vi "OpenVeriStandConnection.vi"(6 "Gateway IP Address (\"\": localhost)":string, 7 "Minimum VeriStand Version (2016)":string="2016", 8 "error in (no error)":errorcluster, 9 "overrides files":path[](array[path]), 10 "System Definition File":path, 11 "VeriStand Test Case in":refnum<class "VeriStandTestCase.lvclass">) -> (0 "error out":errorcluster, 1 "Open Skipped":bool, 3 "VeriStand Test Case out":refnum<class "VeriStandTestCase.lvclass">)   [LabVIEW 2027, in "VeriStandTestCase.lvclass"]
uses:
  VeriStandTestCase.lvclass
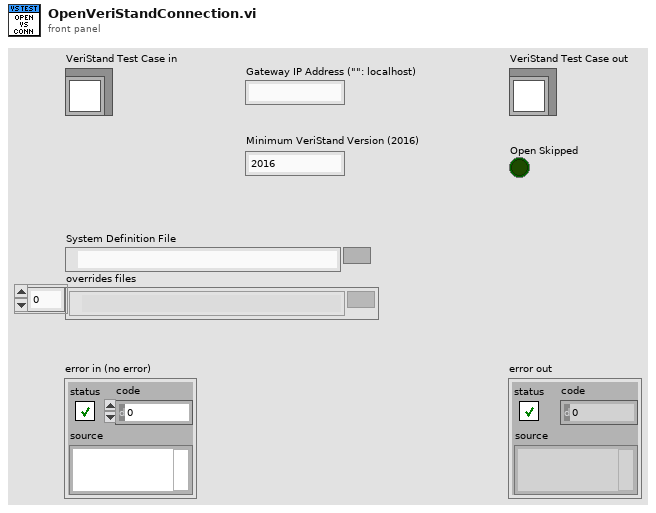
[diagram p1: front panel]
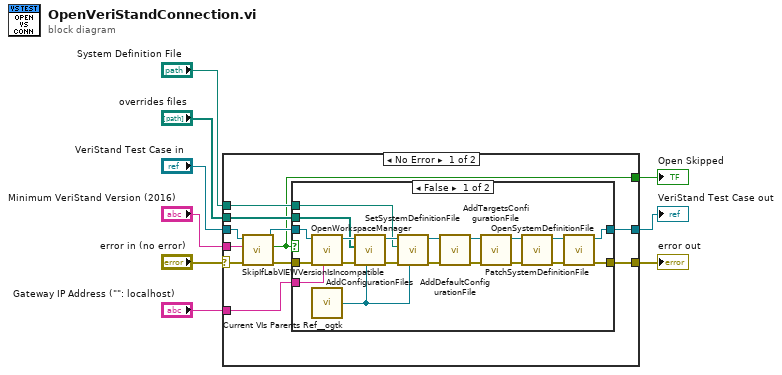
[diagram p0: block diagram]
diagram:
  n1 = case shown="No Error" "error in (no error)" {
    selector: "error in (no error)" -> [w13 w44]
    tunnel: [w19 w44] -> w8
    tunnel: [w20 w43] -> w6
    tunnel: "VeriStand Test Case in" -> [w15 w43]
    tunnel: "System Definition File" -> [w17 _]
    tunnel: "Gateway IP Address (\"\": localhost)" -> [w18 _]
    tunnel: "overrides files" -> [w16 _]
    tunnel: "Minimum VeriStand Version (2016)" -> [w14 _]
    tunnel: [w10 _] -> w1
    frame No Error {
      n2 = call "SkipIfLabVIEWVersionIsIncompatible.vi"("error in (no error)"=w13, "Minimum Version Year (2016)"=w14, "VeriStandTestCase in"=w15) -> ("error out"=w12:errorcluster, "Skipped"=w10:bool, "VeriStandTestCase out"=w11:refnum<class "VeriStandTestCase.lvclass">)  [unwired: 6 in]
      n3 = case shown="False" w10 {
        tunnel: [w40 w42] -> w20
        tunnel: [w39 w41] -> w19
        tunnel: w18 -> [w38 _]
        tunnel: w17 -> [w27 _]
        tunnel: w16 -> [w31 _]
        tunnel: w11 -> [w35 w42]
        tunnel: w12 -> [w34 w41]
        frame False {
          n4 = call "OpenWorkspaceManager.vi"("Gateway IP Address (\"\": localhost)"=w38, "error in (no error)"=w34, "VeriStandTestCase in"=w35) -> ("error out"=w32:errorcluster, "VeriStandTestCase out"=w33:refnum<class "VeriStandTestCase.lvclass">)  [unwired: 7 in]
          n5 = call <userlib>:"Current VIs Parents Ref__ogtk.vi"() -> ("Calling VI's Reference"=w28:refnum<vi>)  [unwired: 2 in]
          n6 = call "AddConfigurationFiles.vi"("path root vi ref (calling vi)"=w28, "error in (no error)"=w32, "configuration files"=w31, "VeriStandTestCase in"=w33) -> ("error out"=w29:errorcluster, "VeriStandTestCase out"=w30:refnum<class "VeriStandTestCase.lvclass">)  [unwired: 6 in]
          n7 = call "SetSystemDefinitionFile.vi"("path root vi ref (calling vi)"=w28, "error in (no error)"=w29, "system definition file"=w27, "VeriStandTestCase in"=w30) -> ("error out"=w26:errorcluster, "VeriStandTestCase out"=w25:refnum<class "VeriStandTestCase.lvclass">)  [unwired: 6 in]
          n8 = call "AddDefaultConfigurationFile.vi"("error in (no error)"=w26, "VeriStandTestCase in"=w25) -> ("error out"=w24:errorcluster, "VeriStandTestCase out"=w21:refnum<class "VeriStandTestCase.lvclass">)  [unwired: 8 in]
          n9 = call "AddTargetsConfigurationFile.vi"("error in (no error)"=w24, "VeriStandTestCase in"=w21) -> ("error out"=w23:errorcluster, "VeriStandTestCase out"=w22:refnum<class "VeriStandTestCase.lvclass">)  [unwired: 8 in]
          n10 = call "PatchSystemDefinitionFile.vi"("error in (no error)"=w23, "VeriStand Test Case in"=w22) -> ("error out"=w37:errorcluster, "VeriStand Test Case out"=w36:refnum<class "VeriStandTestCase.lvclass">)  [unwired: 8 in]
          n11 = call "OpenSystemDefinitionFile.vi"("error in (no error)"=w37, "VeriStand Test Case in"=w36) -> ("error out"=w39:errorcluster, "VeriStand Test Case out"=w40:refnum<class "VeriStandTestCase.lvclass">)  [unwired: 8 in]
        }
        frame True {
        }
      }
    }
    frame Error {
    }
  }
  "error out" <- w8
  "VeriStand Test Case out" <- w6
  "Open Skipped" <- w1
